vi "flush.vi"(8 "error in (no error)":errorcluster, 11 "handle":cluster{}) -> (0 "error out":errorcluster, 2 "function return":i32, 3 "handle out":cluster{})   [LabVIEW 2013, in "buddy.lvlib"]
doc: "EXPORT int buddy_flush(hid_device *handle);"
uses:
  buddy.lvlib
  buddy.dll
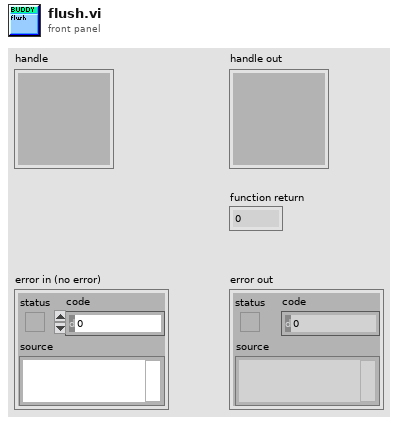
[diagram p1: front panel]
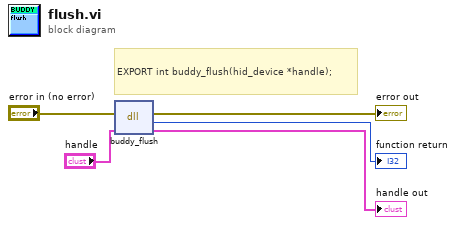
[diagram p0: block diagram]
diagram:
  # "EXPORT int buddy_flush(hid_device *handle);"
  n1 = dll-call lib="C:/Users/shraken/shraken_code/usbhid_buddy/lib/libbuddy/bindings/labview/utility_vi/buddy.*" fn="buddy_flush"(error in="error in (no error)", "handle"="handle") -> (error out=→"error out":errorcluster, →"function return":i32, "handle"=→"handle out":cluster{})  [unwired: 2 in, 1 out]
